vi "Joystick Init.vi"(8 "error in":errorcluster, 11 "JoystickDevice":T1) -> (0 "error out":errorcluster, 3 "Joystick Out":T2)   [LabVIEW 2014]
uses:
  Joystick Info.ctl
  <vilib>/Rock Robotics/WPI/Joystick/WPI_JoystickDevRef.ctl
  <vilib>/Rock Robotics/WPI/Joystick/WPI_JoystickDeviceEnum.ctl
panel:
  in  "Joystick Info":T2
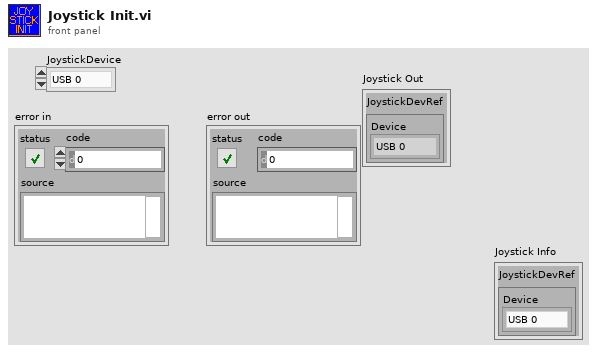
[diagram p1: front panel]
types:
  T1 = typedef "WPI_JoystickDeviceEnum.ctl" = enum16{"USB 0", "USB 1", "USB 2", "USB 3", "USB 4", "USB 5"}
  T2 = typedef "Joystick Info.ctl" = cluster{"JoystickDevRef":T3}
  T3 = typedef "WPI_JoystickDevRef.ctl" = cluster{"Device":T1}
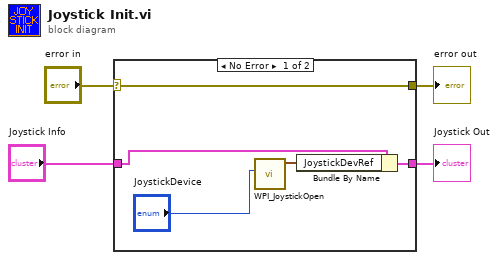
[diagram p0: block diagram]
diagram:
  n1 = case shown="No Error" "error in" {
    selector: "error in" -> [w9 w11]
    tunnel: [w9 w11] -> w3
    tunnel: "Joystick Info" -> [w7 w10]
    tunnel: [w6 w10] -> w1
    frame No Error {
      n2 = call <vilib>:"WPI_JoystickOpen.vi"("JoystickDevice"="JoystickDevice") -> ("JoystickDevRef"=w8:T3)  [unwired: 10 in]
      n3 = Bundle By Name(cluster=w7, "JoystickDevRef"=w8) -> (w6:T2)
    }
    frame Error {
    }
  }
  "error out" <- w3
  "Joystick Out" <- w1
